vi "Read inter-frame delay.vi"(8 "error in (no error)":errorcluster, 11 "MB_ADU_Serial_RTU in":refnum<class "MB_ADU_RTU.lvclass">) -> (0 "error out":errorcluster, 2 "inter-frame delay":u32=2, 3 "MB_ADU_Serial_RTU out":refnum<class "MB_ADU_RTU.lvclass">)   [LabVIEW 2016, in "MB Master.lvlib" / "MB_ADU_RTU.lvclass"]
uses:
  MB_ADU_RTU.lvclass
  MB_ADU_RTU.lvclass/MB_ADU_RTU.ctl
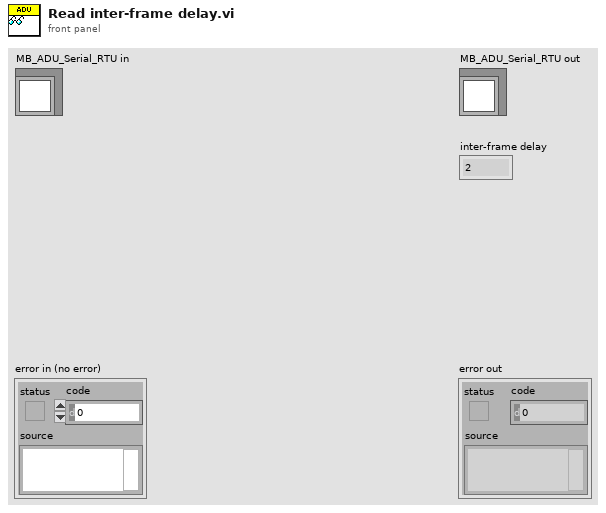
[diagram p1: front panel]
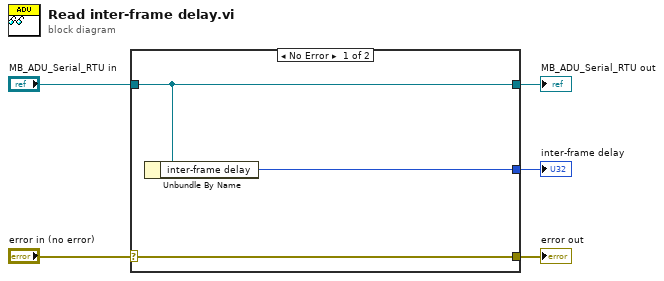
[diagram p0: block diagram]
diagram:
  n1 = case shown="No Error" "error in (no error)" {
    selector: "error in (no error)" -> [w8 w9]
    tunnel: [w8 w9] -> w4
    tunnel: [w7 w10] -> w2
    tunnel: "MB_ADU_Serial_RTU in" -> [w7 w10]
    tunnel: [w6 _] -> w1
    frame No Error {
      n2 = Unbundle By Name(w7) -> ("inter-frame delay"=w6:u32)
    }
    frame Error {
    }
  }
  "error out" <- w4
  "MB_ADU_Serial_RTU out" <- w2
  "inter-frame delay" <- w1
